vi "clear.vi"(8 "error in (no error)":errorcluster, 11 "Bucket in":refnum<class "Bucket.lvclass">) -> (0 "error out":errorcluster, 3 "Bucket out":refnum<class "Bucket.lvclass">)   [LabVIEW 2017, in "Bucket.lvclass"]
uses:
  <userlib>/836-Library/Data_Structures/Bucket/Bucket.lvclass
  <userlib>/836-Library/Data_Structures/Bucket/Bucket.lvclass/Bucket.ctl
  <userlib>/836-Library/Data_Structures/Bucket/Types/KeyValuePair.ctl
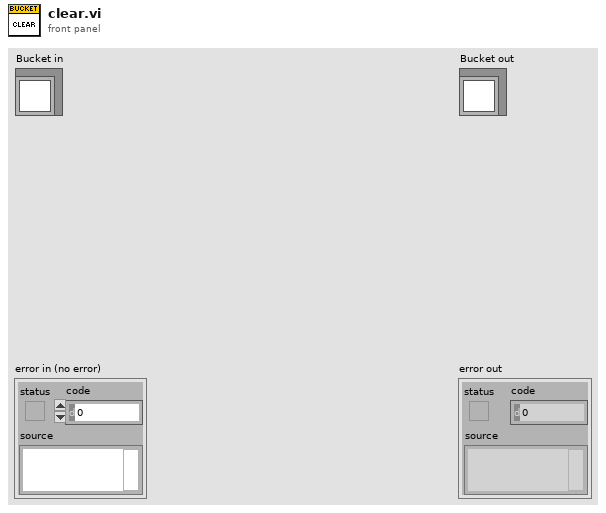
[diagram p1: front panel]
types:
  T1 = typedef "KeyValuePair.ctl" = cluster{"Key":string, "Value":variant}
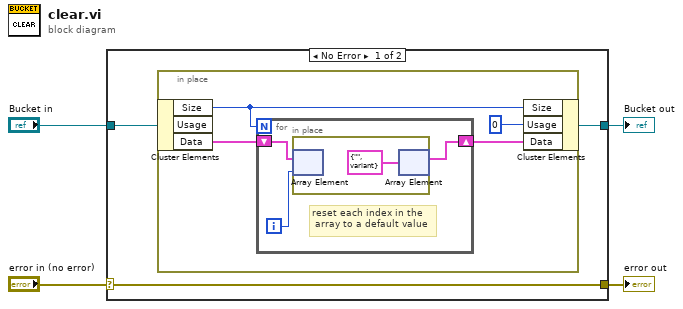
[diagram p0: block diagram]
diagram:
  n1 = case shown="No Error" "error in (no error)" {
    selector: "error in (no error)" -> [w7 w17]
    tunnel: [w7 w17] -> w3
    tunnel: [w5 w16] -> w1
    tunnel: "Bucket in" -> [w6 w16]
    frame No Error {
      n2 = in-place {
        n3 = in-place-cluster #1(w6) -> ("Size"=w8:u32, "Data"=w10:T1[])  [unwired: 1 out]
        n4 = for {
          N: w8 -> [_]
          shift-right: [w12] -> w9
          shift-left: w10 -> [w14]
          i -> [w13]
          # "reset each index in the\n array to a default value"
          n5 = in-place {
            n6 = in-place-array #2(w14, w13) -> ()  [unwired: 1 out]
            n7 = in-place-array #2(T1 {"Key"="", "Value"=variant} ("element")) -> (w12:T1[])  [unwired: 1 out]
          }
        }
        n8 = in-place-cluster #1("Size"=w8, "Usage"=u32 0, "Data"=w9) -> (w5:refnum<class "Bucket.lvclass">)
      }
    }
    frame Error {
    }
  }
  "error out" <- w3
  "Bucket out" <- w1
